vi "Read FlagImpairParams.vi"(8 "error in (no error)":errorcluster, 11 "FlagImpairPluginBase in":refnum<class "FlagImpairPluginBase.lvclass">) -> (0 "error out":errorcluster, 2 "dblFlagImpairParams":dbl[][](array[numeric]), 3 "FlagImpairPluginBase out":refnum<class "FlagImpairPluginBase.lvclass">)   [LabVIEW 2017, in "FlagImpairPlugins.lvlib" / "FlagImpairPluginBase.lvclass"]
uses:
  FlagImpairPluginBase.lvclass
  FlagImpairPluginBase.lvclass/FlagImpairPluginBase.ctl
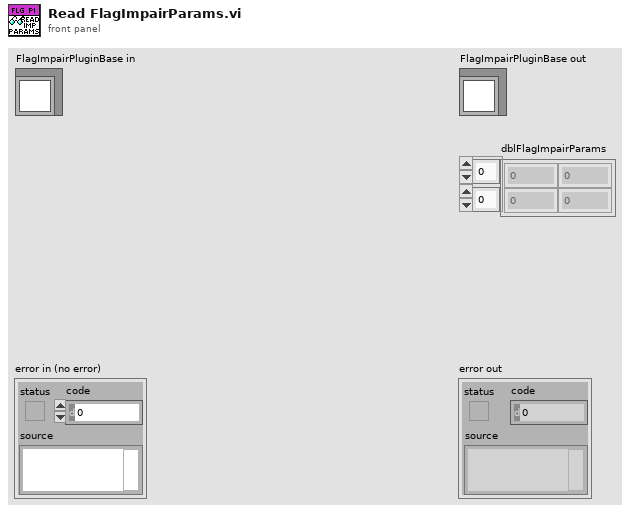
[diagram p1: front panel]
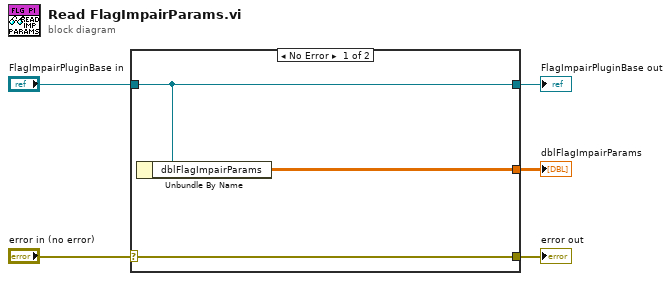
[diagram p0: block diagram]
diagram:
  n1 = case shown="No Error" "error in (no error)" {
    selector: "error in (no error)" -> [w8 w9]
    tunnel: [w8 w9] -> w4
    tunnel: [w7 w10] -> w2
    tunnel: "FlagImpairPluginBase in" -> [w7 w10]
    tunnel: [w6 _] -> w1
    frame No Error {
      n2 = Unbundle By Name(w7) -> ("dblFlagImpairParams"=w6:dbl[][])
    }
    frame Error {
    }
  }
  "error out" <- w4
  "FlagImpairPluginBase out" <- w2
  "dblFlagImpairParams" <- w1
